vi "Load Image as Byte64.vi"(8 "error in (no error)":errorcluster, 11 "path to JPEG file":path=path "C:/batt/IMG_3307.jpg") -> (0 "error out":errorcluster, 3 "Image String":string)   [LabVIEW 2025, in "Battery Prompt.lvlib"]
doc: "Load a JPG file as Byte64 encoded string."
uses:
  Battery Prompt.lvlib
  <vilib>/httpClient/LabVIEWHTTPClient.lvlib
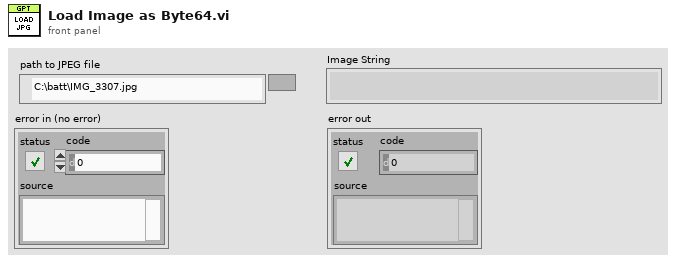
[diagram p1: front panel]
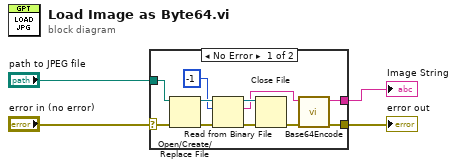
[diagram p0: block diagram]
diagram:
  n1 = case shown="No Error" "error in (no error)" {
    selector: "error in (no error)" -> [w9 w16]
    tunnel: "path to JPEG file" -> [w15 _]
    tunnel: [w10 _] -> w3
    tunnel: [w5 w16] -> w1
    frame No Error {
      n2 = Open/Create/Replace File(file path (use dialog)=w15, error in=w9) -> (refnum out=w14:refnum<file>, error out=w6:errorcluster)  [unwired: 4 in, 1 out]
      n3 = Read from Binary File(8:w6, 10:-1 ("count (1)"), 11:w14) -> (0:w7:errorcluster, 2:w11:string, 3:w12:refnum<file>)  [unwired: 3 in, 1 out]
      n4 = Close File(refnum=w12, error in=w7) -> (error out=w8:errorcluster)  [unwired: 1 out]
      n5 = call <vilib>:"Base64Encode.vi"("error in (no error)"=w8, "buffer in"=w11) -> ("error out"=w5:errorcluster, "encoded string"=w10:string)  [unwired: 8 in]
    }
    frame Error {
    }
  }
  "Image String" <- w3
  "error out" <- w1
